vi "Climb Controller.vi"(8 "error in":errorcluster) -> ()   [LabVIEW 2023]
doc: "This VI executes continuously carrying out the current operation and responding to updates or new operations. It will often contain the timing or control code that is difficult to place directly in TeleOp. This VI generally opens all sensors and motors and isolates the rest of the robot code from knowing how the operations are carried out."
uses:
  <vilib>/Rock Robotics/WPI/Framework/Completion Status.ctl
  Climb Setpoints.ctl
  Climb Operations.ctl
  Support Code/Teleop Util/Climb States.ctl
  <vilib>/Rock Robotics/SystemInterfaces/DIO/FPGA_DIOPWMChannel.ctl
  <vilib>/Rock Robotics/WPI/ThirdParty/REV Robotics/REVLib/Typedef/Spark MAX Idle Mode.ctl
  <vilib>/Rock Robotics/WPI/ThirdParty/REV Robotics/REVLib/Typedef/Spark MAX Control Type.ctl
  <vilib>/Rock Robotics/WPI/ThirdParty/REV Robotics/REVLib/SubVI/Public/SPARK Open Brushless.vi
  <vilib>/Rock Robotics/WPI/ThirdParty/REV Robotics/REVLib/SubVI/Public/SPARK Configure Basic Idle Mode.vi
  <vilib>/Rock Robotics/WPI/ThirdParty/REV Robotics/REVLib/SubVI/Public/SPARK Configure Encoder Conversion Factors.vi
  <vilib>/Rock Robotics/WPI/ThirdParty/REV Robotics/REVLib/SubVI/Public/SPARK Get Encoder Status Position.vi
  Framework/Robot Global Data.vi
  <vilib>/Rock Robotics/Network Tables/NT Write String.vi
  <vilib>/Rock Robotics/Network Tables/NT Write Boolean.vi
panel:
  out "Sensor Position":dbl
  in  "Interactive Values":T1={"Operation"=enum."Reserve", "Setpoint"=0.0, "Duration"=0.0, "Climb States"=enum."Deploy"}
  out "Current\nCmd":string
  in  "Buttons":cluster{"Execute Cmd":bool, "Abort Cmd":bool}
  out "Command Timing":cluster{"Start Time (ms)":u32, "Iterations":i32}
  out "Status":T4
  # "Tip: It may be helpful to observe inputs and sensor values.\nYou may also want to display tuning or debugging controls."
  # "Interactive Command: You may fill in the settings for a command\nand schedule it with the Execute button. You can observe and abort\nany command while fine tuning the code for the controller."
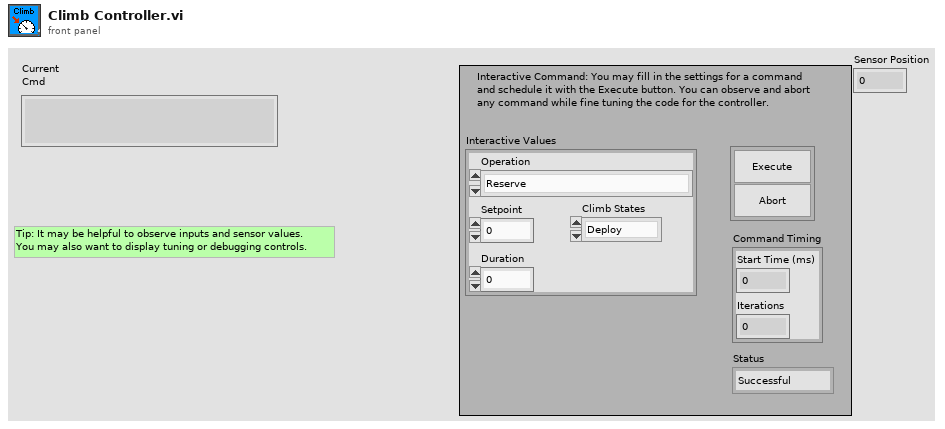
[diagram p1: front panel]
types:
  T1 = typedef "Climb Setpoints.ctl" = cluster{"Operation":T2, "Setpoint":dbl, "Duration":dbl, "Climb States":T3}
  T2 = typedef "Climb Operations.ctl" = enum16{"Reserve", "Read Current", "Immediate"}
  T3 = typedef "Climb States.ctl" = enum16{"Idle", "Deploy", "Undeploy", "Manual Overrides"}
  T4 = typedef "Completion Status.ctl" = enum16{"Successful", "Aborted", "Incomplete"}
  T5 = typedef "Spark MAX Idle Mode.ctl" = enum16{"Coast", "Brake"}
  T6 = typedef "FPGA_DIOPWMChannel.ctl" = enum8{"PWM 0", "PWM 1", "PWM 2", "PWM 3", "PWM 4", "PWM 5", "PWM 6", "PWM 7", "PWM 8", "PWM 9", "PWM MXP 0", "PWM MXP 1", "PWM MXP 2", "PWM MXP 3", "PWM MXP 4", "PWM MXP 5", "PWM MXP 6", "PWM MXP 7", "PWM MXP 8", "PWM MXP 9", "Invalid"}
  T7 = typedef "WPI_MotorControlDeviceRef.ctl" = cluster{"DeviceStatus":errorcluster, "Type":T8, "PWM":cluster{"PWM Channel":T6, "DeadBand":T9}, "CAN":cluster{"Device Number":u8, "SetOutput VI Ref":variant, "GetOutput VI Ref":variant, "Enable VI Ref":variant, "Disable VI Ref":variant, "Data":variant}, "Invert":bool, "DIO PWM":cluster{"PWM \"Enable\" Channel":T6, "DIOChannel":T10, "PWM Rate":dbl}}
  T8 = typedef "WPI_MotorControlType.ctl" = enum16{"PWM", "CAN", "DIO PWM"}
  T9 = typedef "WPI_PWMDeadband.ctl" = cluster{"Name":string, "maxPositivePwm":i32, "minPositivePwm":i32, "centerPwm":i32, "maxNegativePwm":i32, "minNegativePwm":i32, "angularRange":u16}
  T10 = typedef "FPGA_DIOChannel.ctl" = enum8{"DIO 0", "DIO 1", "DIO 2", "DIO 3", "DIO 4", "DIO 5", "DIO 6", "DIO 7", "DIO 8", "DIO 9", "DIO MXP 0", "DIO MXP 1", "DIO MXP 2", "DIO MXP 3", "DIO MXP 4", "DIO MXP 5", "DIO MXP 6", "DIO MXP 7", "DIO MXP 8", "DIO MXP 9", "DIO MXP 10", "DIO MXP 11", "DIO MXP 12", "DIO MXP 13", "DIO MXP 14", "DIO MXP 15", "SPI Port CS1", "SPI Port CS2", "SPI Port CS3", "SPI Port MISO", "SPI Port MOSI", "Invalid"}
  T11 = typedef "WPI_ServoDeviceRef.ctl" = cluster{"DeviceStatus":errorcluster, "PWM Channel":T6, "DeadBand":T9}
  T12 = typedef "Command Status Info.ctl" = cluster{"Name":string, "Status":T4, "notifier out":T13}
  T13 = typedef "Completion Notifier.ctl" = refnum<notifier>
  T14 = cluster{"Current Command":T1, "Command Timing":cluster{"Start Time (ms)":u32, "Iterations":i32}, "Command Arguments":cluster{"Command Info":T12, "Description":string, "Default Command":T1, "queue out":refnum<queue>, "Subsystem Name":string}}
  T15 = typedef "Spark MAX Control Type.ctl" = enum16{"Percent VBus", "Voltage", "Velocity", "Position", "Smart Motion", "Current", "Smart Velocity", "MAXMotion Position", "MAXMotion Velocity"}
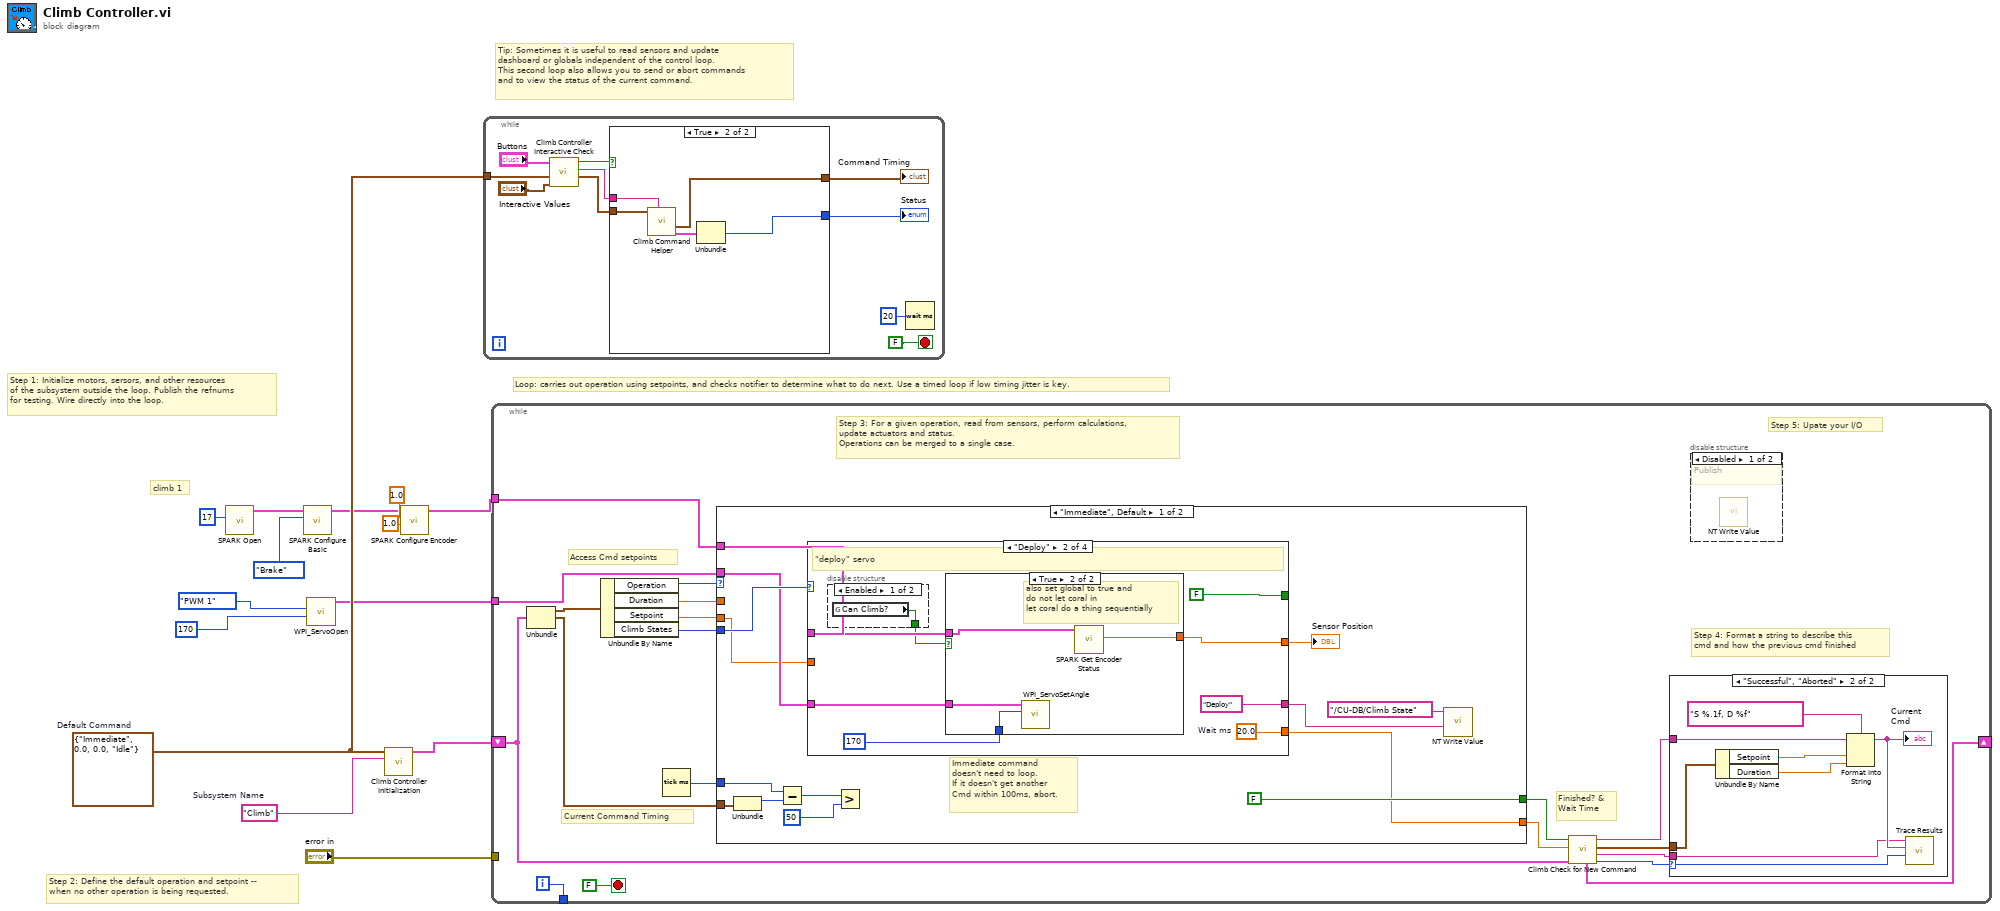
[diagram p0: block diagram]
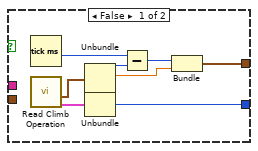
[diagram p2: hidden frame]
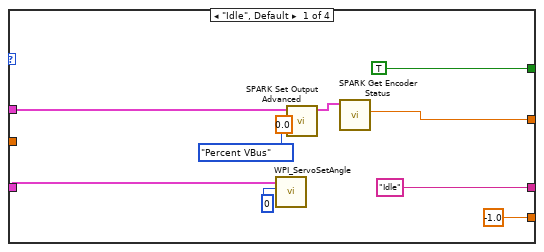
[diagram p5: hidden frame]
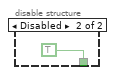
[diagram p6: hidden frame]
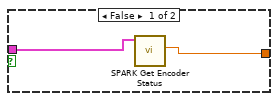
[diagram p7: hidden frame]
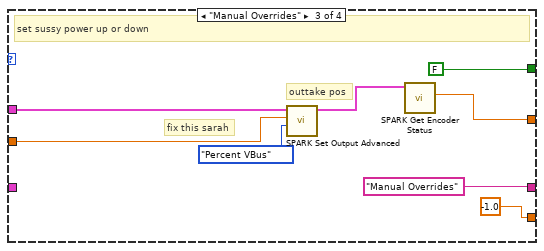
[diagram p8: hidden frame]
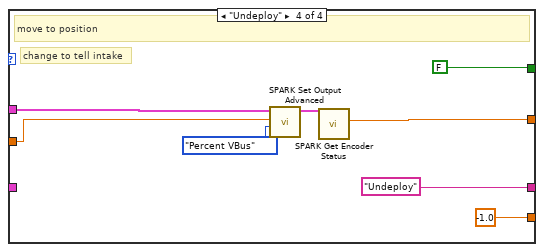
[diagram p9: hidden frame]
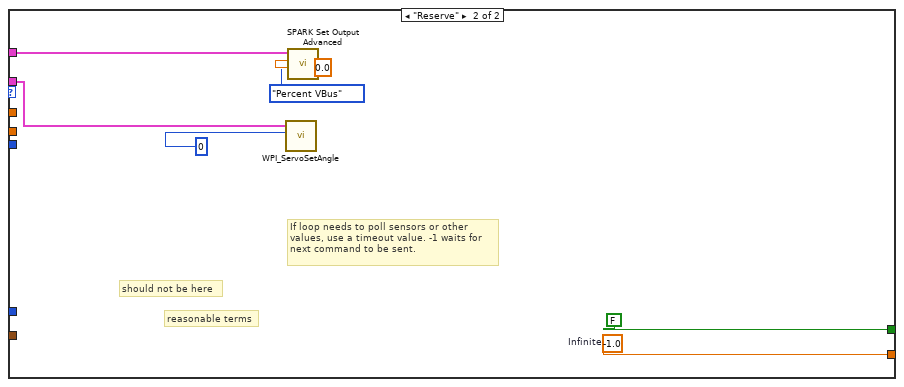
[diagram p10: hidden frame]
diagram:
  w11 = T1 {"Operation"=enum."Immediate", "Setpoint"=0.0, "Duration"=0.0, "Climb States"=enum."Idle"}  # Default Command
  w12 = "Climb"  # Subsystem Name
  # "climb 1"
  # "Tip: Sometimes it is useful to read sensors and update\ndashboard or globals independent of the control loop.\nThis second loop also allows you to send or abort commands\nand to view the status of the current command."
  # "Step 2: Define the default operation and setpoint --\nwhen no other operation is being requested."
  # "Step 1: Initialize motors, sersors, and other resources\nof the subsystem outside the loop. Publish the refnums\nfor testing. Wire directly into the loop."
  # "Loop: carries out operation using setpoints, and checks notifier to determine what to do next. Use a timed loop if low timing jitter is key."
  n1 = call-poly <vilib>:"SPARK Open.vi"("Device Number"=u8 17) -> ("MotorControlDeviceRef"=w1:T7)  [unwired: 9 in, 1 out]
  n2 = call-poly <vilib>:"SPARK Configure Basic.vi"("Idle Mode"=Spark_MAX_Idle_Mode."Brake", "MotorControlDeviceRef in"=w1) -> ("MotorControlDeviceRef out"=w2:T7)  [unwired: 8 in, 1 out]
  n3 = call <vilib>:"WPI_ServoOpen.vi"("Angular Range"=u16 170, "PWM Channel"=FPGA_DIOPWMChannel."PWM 1") -> ("ServoDeviceRef"=w7:T11)  [unwired: 8 in, 1 out]
  n4 = call "Climb Controller Initialization.vi"("Subsystem Name"=w12, "Default Command"=w11) -> ("Current Command"=w13:T14)  [unwired: 9 in]
  n5 = call-poly <vilib>:"SPARK Configure Encoder.vi"("Velocity Conversion Factor"=1.0, "Position Conversion Factor"=1.0, "MotorControlDeviceRef in"=w2) -> ("MotorControlDeviceRef out"=w3:T7)  [unwired: 7 in, 1 out]
  n6 = while {
    tunnel: w11 -> [w21]
    stop <- FALSE stop-if-true
    n7 = call "Climb Controller Interactive Check.vi"("Interactive Command in"="Interactive Values", "Default Command"=w21, "Buttons"="Buttons") -> ("Interactive Command out"=w18:T1, "Trace String"=w19:string, "Schedule"=w20:bool)  [unwired: 6 in]
    n8 = case shown="True" w20 {
      tunnel: [w32 w37] -> w17
      tunnel: w18 -> [_ w35]
      tunnel: [w28 w33] -> w16
      tunnel: w19 -> [_ w36]
      frame False {
        n9 = Tick Count (ms)() -> (millisecond timer value=w27:u32)
        n10 = call "Read Climb Operation.vi"() -> ("Command Info"=w25:T12, "SubSystem Data"=w26:T1)  [unwired: 9 in, 1 out]
        n11 = Unbundle(w26) -> ("Operation"=w31:T2, "Setpoint"=w29:dbl)  [unwired: 2 out]
        n12 = Unbundle(w25) -> ("Status"=w32:T4)  [unwired: 2 out]
        n13 = Subtract(x=w27, y=w31) -> (x-y=w30:u32)
        n14 = Bundle(w30, "Setpoint"=w29) -> (w28:cluster{u32, "Setpoint":dbl})  [unwired: 1 in]
      }
      frame True {
        n15 = call "Climb Command Helper.vi"("Description"=w36, "SubSystem Data"=w35) -> ("Command Info Out"=w34:T12, "Command Timing"=w33:cluster{"Start Time (ms)":u32, "Iterations":i32})  [unwired: 7 in, 1 out]
        n16 = Unbundle(w34) -> ("Status"=w37:T4)  [unwired: 2 out]
      }
    }
    "Status" <- w17
    "Command Timing" <- w16
    n17 = Wait (ms)(milliseconds to wait=u32 20) -> ()  [unwired: 1 out]
  }
  n18 = while {
    shift-right: [w48] -> _
    shift-left: w13 -> [w41]
    tunnel: [w55] -> _
    tunnel: "error in" -> [_]
    tunnel: w7 -> [w39]
    tunnel: w3 -> [w38]
    i -> [w55]
    stop <- FALSE stop-if-true
    # "Step 5: Upate your I/O"
    # "Step 4: Format a string to describe this\ncmd and how the previous cmd finished"
    # "Current Command Timing"
    # "Access Cmd setpoints"
    # "Finished? &\nWait Time"
    # "Step 3: For a given operation, read from sensors, perform calculations,\nupdate actuators and status.\nOperations can be merged to a single case."
    n19 = Unbundle(w41) -> ("Current Command"=w54:T1, "Command Timing"=w50:cluster{"Start Time (ms)":u32, "Iterations":i32})  [unwired: 1 out]
    n20 = Unbundle By Name(w54) -> ("Operation"=w53:T2, "Duration"=w52:dbl, "Setpoint"=w49:dbl, "Climb States"=w40:T3)
    n21 = Tick Count (ms)() -> (millisecond timer value=w51:u32)
    n22 = case shown="\"Immediate\", Default" w53 {
      tunnel: [w65 w127] -> w46
      tunnel: [FALSE ("ignore previous (F)") FALSE ("ignore previous (F)")] -> w47
      tunnel: w50 -> [w75 _]
      tunnel: w52 -> [_ _]
      tunnel: w51 -> [w74 _]
      tunnel: w49 -> [w69 _]
      tunnel: w40 -> [w72 _]
      tunnel: w38 -> [w71 w123]
      tunnel: w39 -> [w70 w122]
      frame "Immediate", Default {
        # "Immediate command\ndoesn't need to loop.\nIf it doesn't get another\nCmd within 100ms, abort."
        n23 = Unbundle(w75) -> ("Start Time (ms)"=w78:u32)  [unwired: 1 out]
        n24 = Subtract(x=w74, y=w78) -> (x-y=w77:u32)
        n25 = case shown="\"Deploy\"" w72 {
          tunnel: w71 -> [w86 w96 w111 w120]
          tunnel: w70 -> [w84 w95 _ _]
          tunnel: [TRUE ("Can Return?") FALSE ("Can Return?") FALSE ("Can Return?") FALSE ("Can Return?")] -> _
          tunnel: [w81 w93 w108 w118] -> w68
          tunnel: w69 -> [_ _ w107 w115]
          tunnel: ["Idle" "Deploy" "Manual Overrides" "Undeploy"] -> w66
          tunnel: [-1.0 ("Wait ms") w90 -1.0 ("Wait ms") -1.0 ("Wait ms")] -> w65
          frame "Idle", Default {
            n26 = call <vilib>:"WPI_ServoSetAngle.vi"("Angle"=0, "ServoDeviceRef"=w84) -> ()  [unwired: 8 in, 2 out]
            n27 = call <vilib>:"SPARK Set Output Advanced.vi"("Control Mode"=Spark_MAX_Control_Type."Percent VBus", "Setpoint"=0.0, "MotorControlDevRef"=w86) -> ("MotorControlDevRef"=w82:T7)  [unwired: 7 in, 1 out]
            n28 = call-poly <vilib>:"SPARK Get Encoder Status.vi"("MotorControlDevRef in"=w82) -> ("Sensor Position"=w81:dbl)  [unwired: 7 in, 3 out]
          }
          frame "Deploy" {
            w90 = 20.0  # Wait ms
            # "\"deploy\" servo"
            n29 = disable-structure shown="Enabled" {
              disable-tunnel: [w97 TRUE ("Can Climb?")] -> w92
              frame Enabled {
                n30 = global read "Robot Global Data.vi" "Can Climb?"() -> (w97:bool)
              }
              frame Disabled {
              }
            }
            n31 = case shown="True" w92 {
              tunnel: w96 -> [w99 w104]
              tunnel: w95 -> [_ w103]
              tunnel: 170 ("Angle") -> [_ w102]
              tunnel: [w100 w101] -> w93
              frame False {
                n32 = call-poly <vilib>:"SPARK Get Encoder Status.vi"("MotorControlDevRef in"=w99) -> ("Sensor Position"=w100:dbl)  [unwired: 7 in, 3 out]
              }
              frame True {
                # "also set global to true and \ndo not let coral in\nlet coral do a thing sequentially"
                n33 = call <vilib>:"WPI_ServoSetAngle.vi"("Angle"=w102, "ServoDeviceRef"=w103) -> ()  [unwired: 8 in, 2 out]
                n34 = call-poly <vilib>:"SPARK Get Encoder Status.vi"("MotorControlDevRef in"=w104) -> ("Sensor Position"=w101:dbl)  [unwired: 7 in, 3 out]
              }
            }
          }
          frame "Manual Overrides" {
            # "fix this sarah"
            # "outtake pos"
            # "set sussy power up or down"
            n35 = call <vilib>:"SPARK Set Output Advanced.vi"("Control Mode"=Spark_MAX_Control_Type."Percent VBus", "Setpoint"=w107, "MotorControlDevRef"=w111) -> ("MotorControlDevRef"=w109:T7)  [unwired: 7 in, 1 out]
            n36 = call-poly <vilib>:"SPARK Get Encoder Status.vi"("MotorControlDevRef in"=w109) -> ("Sensor Position"=w108:dbl)  [unwired: 7 in, 3 out]
          }
          frame "Undeploy" {
            # "change to tell intake"
            # "move to position"
            n37 = call <vilib>:"SPARK Set Output Advanced.vi"("Control Mode"=Spark_MAX_Control_Type."Percent VBus", "Setpoint"=w115, "MotorControlDevRef"=w120) -> ("MotorControlDevRef"=w116:T7)  [unwired: 7 in, 1 out]
            n38 = call-poly <vilib>:"SPARK Get Encoder Status.vi"("MotorControlDevRef in"=w116) -> ("Sensor Position"=w118:dbl)  [unwired: 7 in, 3 out]
          }
        }
        "Sensor Position" <- w68
        n39 = Greater?(x=w77, y=u8 50 ("Left Motor")) -> ()  [unwired: 1 out]
        n40 = call-poly <vilib>:"NT Write Value.vi"("value"=w66, "name"="/CU-DB/Climb State") -> ()  [unwired: 9 in, 1 out]
      }
      frame "Reserve" {
        w127 = -1.0  # Infinite
        # "reasonable terms"
        # "should not be here"
        # "If loop needs to poll sensors or other\nvalues, use a timeout value. -1 waits for\nnext command to be sent."
        n41 = call <vilib>:"WPI_ServoSetAngle.vi"("Angle"=0, "ServoDeviceRef"=w122) -> ()  [unwired: 8 in, 2 out]
        n42 = call <vilib>:"SPARK Set Output Advanced.vi"("Control Mode"=Spark_MAX_Control_Type."Percent VBus", "Setpoint"=0.0, "MotorControlDevRef"=w123) -> ()  [unwired: 7 in, 2 out]
      }
    }
    n43 = call "Climb Check for New Command.vi"("Current Command"=w41, "Wait time (ms)"=w46, "Finished?"=w47) -> ("Completion"=w42:T4, "Subsystem Name"=w43:string, "Current Command"=w44:T1, "Initial Trace String"=w45:string, "NextCommand"=w48:T14)  [unwired: 4 in]
    n44 = case shown="\"Successful\", \"Aborted\"" w42 {
      selector: w42 -> [_ w64]
      tunnel: w45 -> [_ w60]
      tunnel: w44 -> [_ w61]
      tunnel: w43 -> [_ w57]
      frame "Incomplete", Default {
        # "Continuing current command"
      }
      frame "Successful", "Aborted" {
        # "Report and setup for next command"
        n45 = Unbundle By Name(w61) -> ("Setpoint"=w63:dbl, "Duration"=w58:dbl)
        n46 = Format Into String(format string="S %.1f, D %f", initial string=w60, w63, w58) -> (resulting string=w59:string)  [unwired: 1 in, 1 out]
        "Current\nCmd" <- w59
        n47 = call <vilib>:"Trace Results.vi"("Status of previous command"=w64, "Description"=w59, "Subsystem"=w57) -> ()  [unwired: 9 in]
      }
    }
    n48 = disable-structure shown="Disabled" {
      frame Disabled {
        # "Publish"
        n49 = call-poly <vilib>:"NT Write Value.vi"() -> ()  [unwired: 11 in, 1 out]
      }
      frame Enabled {
      }
    }
  }
